vi "Set Version Information.vi"(8 "error in (no error)":errorcluster, 10 "Version Information":T1, 11 "NI_AB_API_Targetfile in":refnum<class "NI_AB_API_Targetfile.lvclass">) -> (0 "error out":errorcluster, 3 "NI_AB_API_Targetfile out":refnum<class "NI_AB_API_Targetfile.lvclass">)   [LabVIEW 2020, in "NI_AB_API_Targetfile.lvclass"]
uses:
  <vilib>/AppBuilder/AB_API/Targetfile/NI_AB_API_Targetfile.lvclass
  e:/builds/penguin/labview/branches/2020/dev/dist/vi.lib/AppBuilder/AB_API/Build/NI_AB_API_Build.lvclass
  <vilib>/AppBuilder/AB_API/common/AB_API Version Information.ctl
  <vilib>/AppBuilder/AB_Classes/TargetFile/AB_Targetfile.lvclass
  e:/builds/penguin/labview/branches/2020/dev/dist/vi.lib/AppBuilder/AB_Classes/Build/AB_Build.lvclass
  <vilib>/AppBuilder/AB_API/Targetfile/NI_AB_API_Targetfile.lvclass/NI_AB_API_Targetfile.ctl
  <vilib>/AppBuilder/AB_API/Build/NI_AB_API_Build.lvclass
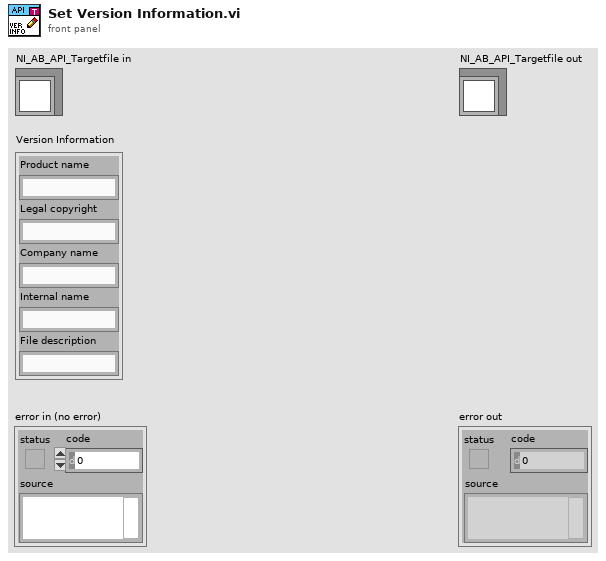
[diagram p1: front panel]
types:
  T1 = typedef "AB_API Version Information.ctl" = cluster{"Product name":string, "Legal copyright":string, "Company name":string, "Internal name":string, "File description":string}
  T2 = typedef "AB_Targetfile.ctl" = cluster{"targetfileName":string, "targetfileGUID":string, "enableDebugging":bool, "versionInfo":cluster{"productName":string, "legalCopyright":string, "companyName":string, "internalName":string, "fileDescription":string}, "eng_consolidatedTypeInfo":string, "fastFileFormat":bool, "eng_LEIFBuildData":u32, "versionIndependent":bool}
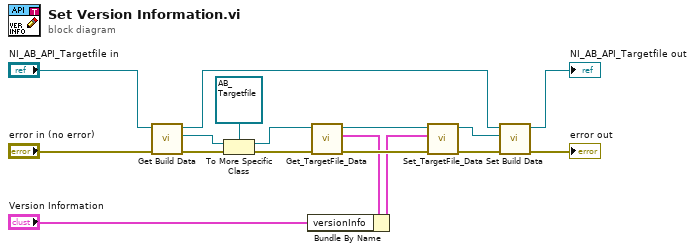
[diagram p0: block diagram]
diagram:
  n1 = call <vilib>:"Get Build Data.vi"("error in (no error)"="error in (no error)", "NI_AB_API_Build in"="NI_AB_API_Targetfile in") -> ("error out"=w9:errorcluster, "AB_Build.lvclass"=w8:refnum<class "AB_Build.lvclass">, "NI_AB_API_Build out"=w6:refnum<class "NI_AB_API_Targetfile.lvclass">)  [unwired: 7 in]
  n2 = To More Specific Class(target class=refnum<class "AB_Targetfile.lvclass"> refnum ("AB_Targetfile in"), reference=w8, error in=w9) -> (specific class reference=w3:refnum<class "AB_Targetfile.lvclass">, error out=w2:errorcluster)
  n3 = call <vilib>:"Get_TargetFile_Data.vi"("error in (no error)"=w2, "AB_Targetfile in"=w3) -> ("error out"=w13:errorcluster, "data"=w11:T2, "AB_Targetfile out"=w12:refnum<class "AB_Targetfile.lvclass">)  [unwired: 7 in]
  n4 = Bundle By Name(cluster=w11, "versionInfo"="Version Information") -> (w10:T2)
  n5 = call <vilib>:"Set_TargetFile_Data.vi"("error in (no error)"=w13, "data"=w10, "AB_Targetfile in"=w12) -> ("error out"=w5:errorcluster, "AB_Targetfile out"=w4:refnum<class "AB_Targetfile.lvclass">)  [unwired: 7 in]
  n6 = call <vilib>:"Set Build Data.vi"("error in (no error)"=w5, "AB_Build.lvclass"=w4, "NI_AB_API_Build in"=w6) -> ("error out"=→"error out":errorcluster, "NI_AB_API_Build out"=→"NI_AB_API_Targetfile out":refnum<class "NI_AB_API_Targetfile.lvclass">)  [unwired: 7 in]
